vi "GetParent.vi"(8 "error in (no error)":errorcluster, 10 "Tag":string, 11 "TreeControl in":refnum<vi>) -> (0 "error out":errorcluster, 1 "Child Index":i32, 2 "Parent Tag":string, 3 "TreeControl out":refnum<vi>)   [LabVIEW 2021, in "TreeControlLib.lvlib"]
uses:
  TreeControlLib.lvlib
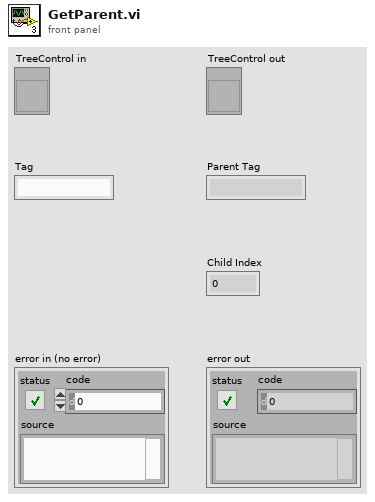
[diagram p1: front panel]
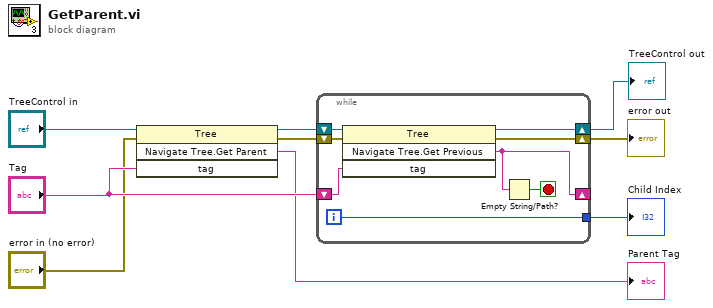
[diagram p0: block diagram]
diagram:
  n1 = invoke class="Tree" method="Navigate Tree.Get Parent"(reference="TreeControl in", error in="error in (no error)", "tag"="Tag") -> (reference out=w8:refnum<vi>, error out=w3:errorcluster, "Navigate Tree:Get Parent"=→"Parent Tag":string)  [unwired: 1 in, 1 out]
  n2 = while {
    shift-right: [w15] -> _
    shift-left: "Tag" -> [w16]
    tunnel: [w13] -> w5
    shift-right: [w11] -> w2
    shift-left: w3 -> [w12]
    shift-right: [w10] -> w1
    shift-left: w8 -> [w17]
    i -> [w13]
    stop <- w14 stop-if-true
    n3 = invoke class="Tree" method="Navigate Tree.Get Previous"(reference=w17, error in=w12, "tag"=w16) -> (reference out=w10:refnum<vi>, error out=w11:errorcluster, "Navigate Tree:Get Previous"=w15:string)  [unwired: 1 in, 1 out]
    n4 = Empty String/Path?(string/path=w15) -> (empty?=w14:bool)
  }
  "Child Index" <- w5
  "error out" <- w2
  "TreeControl out" <- w1
